vi "GeoData.vi"() -> ()   [LabVIEW 2017] (continued)
H1\n93203\t6029\tArvin\tCA\tKern County\tH1\n93250\t6029\tMc farland\tCA\tKern County\tH1\n93206\t6029\tButtonwillow\tCA\tKern County\tH1\n93384\t6029\tBakersfield\tCA\tKern County\tH1\n93502\t6029\tMojave\tCA\tKern County\tH1\n93255\t6029\tOnyx\tCA\tKern County\tH1\n93226\t6029\tGlennville\tCA\tKern County\tH1\n93528\t6029\tJohannesburg\tCA\tKern County\tH1\n93301\t6029\tBakersfield\tCA\tKern County\tH1\n93308\t6029\tBakersfield\tCA\tKern County\tH1\n93305\t6029\tBakersfield\tCA\tKern County\tH1\n93302\t6029\tBakersfield\tCA\tKern County\tH1\n93505\t6029\tCalifornia city\tCA\tKern County\tH1\n93561\t6029\tTehachapi\tCA\tKern County\tH1\n93461\t6029\tShandon\tCA\tKern County\tH1\n93268\t6029\tTaft\tCA\tKern County\tH1\n93241\t6029\tLamont\tCA\tKern County\tH1\n93263\t6029\tShafter\tCA\tKern County\tH1\n93518\t6029\tCaliente\tCA\tKern County\tH1\n93249\t6029\tLost hills\tCA\tKern County\tH1\n93303\t6029\tBakersfield\tCA\tKern County\tH1\n93222\t6029\tPine mountain club\tCA\tKern County\tH1\n93312\t6029\tBakersfield\tCA\tKern County\tH1\n93501\t6029\tMojave\tCA\tKern County\tH1\n93523\t6029\tEdwards\tCA\tKern County\tH1\n93240\t6029\tLake isabella\tCA\tKern County\tH1\n93238\t6029\tKernville\tCA\tKern County\tH1\n93251\t6029\tMc kittrick\tCA\tKern County\tH1\n93313\t6029\tBakersfield\tCA\tKern County\tH1\n93536\t6029\tLancaster\tCA\tKern County\tH1\n93516\t6029\tBoron\tCA\tKern County\tH1\n93219\t6029\tEarlimart\tCA\tKern County\tH1\n93224\t6029\tFellows\tCA\tKern County\tH1\n93252\t6029\tMaricopa\tCA\tKern County\tH1\n93554\t6029\tRandsburg\tCA\tKern County\tH1\n93309\t6029\tBakersfield\tCA\tKern County\tH1\n93387\t6029\tBakersfield\tCA\tKern County\tH1\n93524\t6029\tEdwards\tCA\tKern County\tH1\n93531\t6029\tKeene\tCA\tKern County\tH1\n93276\t6029\tTupman\tCA\tKern County\tH1\n93314\t6029\tBakersfield\tCA\tKern County\tH1\n93527\t6029\tInyokern\tCA\tKern County\tH1\n93225\t6029\tFrazier park\tCA\tKern County\tH1\n93280\t6029\tWasco\tCA\tKern County\tH1\n93389\t6029\tBakersfield\tCA\tKern County\tH1\n93239\t6031\tKettleman city\tCA\tKings County\tH1\n93266\t6031\tStratford\tCA\tKings County\tH1\n93656\t6031\tRiverdale\tCA\tKings County\tH1\n93274\t6031\tTulare\tCA\tKings County\tH1\n93246\t6031\tLemoore\tCA\tKings County\tH1\n93204\t6031\tAvenal\tCA\tKings County\tH1\n93230\t6031\tHanford\tCA\tKings County\tH1\n93631\t6031\tKingsburg\tCA\tKings County\tH1\n93212\t6031\tCorcoran\tCA\tKings County\tH1\n93202\t6031\tArmona\tCA\tKings County\tH1\n93232\t6031\tHanford\tCA\tKings County\tH1\n93245\t6031\tLemoore\tCA\tKings County\tH1\n93242\t6031\tLaton\tCA\tKings County\tH1\n95457\t6033\tLower lake\tCA\tLake County\tH1\n95423\t6033\tClearlake oaks\tCA\tLake County\tH1\n95424\t6033\tClearlake park\tCA\tLake County\tH1\n95451\t6033\tKelseyville\tCA\tLake County\tH1\n95467\t6033\tHidden valley lake\tCA\tLake County\tH1\n95485\t6033\tUpper lake\tCA\tLake County\tH1\n95422\t6033\tClearlake\tCA\tLake County\tH1\n95458\t6033\tLucerne\tCA\tLake County\tH1\n95453\t6033\tLakeport\tCA\tLake County\tH1\n95461\t6033\tMiddletown\tCA\tLake County\tH1\n95435\t6033\tFinley\tCA\tLake County\tH1\n95464\t6033\tNice\tCA\tLake County\tH1\n95443\t6033\tGlenhaven\tCA\tLake County\tH1\n95426\t6033\tCobb\tCA\tLake County\tH1\n95469\t6033\tPotter valley\tCA\tLake County\tH1\n95493\t6033\tWitter springs\tCA\tLake County\tH1\n96114\t6035\tJanesville\tCA\tLassen County\tH1\n96121\t6035\tMilford\tCA\tLassen County\tH1\n96128\t6035\tStandish\tCA\tLassen County\tH1\n96132\t6035\tTermo\tCA\tLassen County\tH1\n96136\t6035\tWendel\tCA\tLassen County\tH1\n96119\t6035\tMadeline\tCA\tLassen County\tH1\n96109\t6035\tDoyle\tCA\tLassen County\tH1\n96009\t6035\tBieber\tCA\tLassen County\tH1\n96127\t6035\tSusanville\tCA\tLassen County\tH1\n96117\t6035\tLitchfield\tCA\tLassen County\tH1\n96130\t6035\tSusanville\tCA\tLassen County\tH1\n96056\t6035\tMcarthur\tCA\tLassen County\tH1\n96068\t6035\tNubieber\tCA\tLassen County\tH1\n96137\t6035\tWestwood\tCA\tLassen County\tH1\n96113\t6035\tHerlong\tCA\tLassen County\tH1\n96123\t6035\tRavendale\tCA\tLassen County\tH1\n90013\t6037\tLos angeles\tCA\tLos Angeles County\tH1\n90232\t6037\tCulver city\tCA\tLos Angeles County\tH1\n90067\t6037\tLos angeles\tCA\tLos Angeles County\tH1\n90254\t6037\tHermosa beach\tCA\tLos Angeles County\tH1\n90305\t6037\tInglewood\tCA\tLos Angeles County\tH1\n90409\t6037\tSanta monica\tCA\tLos Angeles County\tH1\n90723\t6037\tParamount\tCA\tLos Angeles County\tH1\n90749\t6037\tCarson\tCA\tLos Angeles County\tH1\n90710\t6037\tHarbor city\tCA\tLos Angeles County\tH1\n90507\t6037\tTorrance\tCA\tLos Angeles County\tH1\n90043\t6037\tLos angeles\tCA\tLos Angeles County\tH1\n90059\t6037\tLos angeles\tCA\tLos Angeles County\tH1\n91101\t6037\tPasadena\tCA\tLos Angeles County\tH1\n91202\t6037\tGlendale\tCA\tLos Angeles County\tH1\n91008\t6037\tDuarte\tCA\tLos Angeles County\tH1\n91304\t6037\tCanoga park\tCA\tLos Angeles County\tH1\n91328\t6037\tNorthridge\tCA\tLos Angeles County\tH1\n91307\t6037\tWest hills\tCA\tLos Angeles County\tH1\n93560\t6037\tRosamond\tCA\tLos Angeles County\tH1\n91384\t6037\tCastaic\tCA\tLos Angeles County\tH1\n91405\t6037\tVan nuys\tCA\tLos Angeles County\tH1\n91345\t6037\tMission hills\tCA\tLos Angeles County\tH1\n91350\t6037\tSanta clarita\tCA\tLos Angeles County\tH1\n90670\t6037\tSanta fe springs\tCA\tLos Angeles County\tH1\n90660\t6037\tPico rivera\tCA\tLos Angeles County\tH1\n90638\t6037\tLa mirada\tCA\tLos Angeles County\tH1\n91711\t6037\tClaremont\tCA\tLos Angeles County\tH1\n91755\t6037\tMonterey park\tCA\tLos Angeles County\tH1\n91791\t6037\tWest covina\tCA\tLos Angeles County\tH1\n91770\t6037\tRosemead\tCA\tLos Angeles County\tH1\n91780\t6037\tTemple city\tCA\tLos Angeles County\tH1\n90051\t6037\tLos angeles\tCA\tLos Angeles County\tH1\n91025\t6037\tSierra madre\tCA\tLos Angeles County\tH1\n91778\t6037\tSan gabriel\tCA\tLos Angeles County\tH1\n91614\t6037\tStudio city\tCA\tLos Angeles County\tH1\n91066\t6037\tArcadia\tCA\tLos Angeles County\tH1\n91327\t6037\tNorthridge\tCA\tLos Angeles County\tH1\n93243\t6037\tLebec\tCA\tLos Angeles County\tH1\n91407\t6037\tVan nuys\tCA\tLos Angeles County\tH1\n90310\t6037\tInglewood\tCA\tLos Angeles County\tH1\n91603\t6037\tNorth hollywood\tCA\tLos Angeles County\tH1\n90306\t6037\tInglewood\tCA\tLos Angeles County\tH1\n91021\t6037\tMontrose\tCA\tLos Angeles County\tH1\n90822\t6037\tLong beach\tCA\tLos Angeles County\tH1\n91123\t6037\tPasadena\tCA\tLos Angeles County\tH1\n91129\t6037\tPasadena\tCA\tLos Angeles County\tH1\n91804\t6037\tAlhambra\tCA\tLos Angeles County\tH1\n90017\t6037\tLos angeles\tCA\tLos Angeles County\tH1\n90021\t6037\tLos angeles\tCA\tLos Angeles County\tH1\n90210\t6037\tBeverly hills\tCA\tLos Angeles County\tH1\n90071\t6037\tLos angeles\tCA\tLos Angeles County\tH1\n90266\t6037\tManhattan beach\tCA\tLos Angeles County\tH1\n90265\t6037\tMalibu\tCA\tLos Angeles County\tH1\n90401\t6037\tSanta monica\tCA\tLos Angeles County\tH1\n90503\t6037\tTorrance\tCA\tLos Angeles County\tH1\n90267\t6037\tManhattan beach\tCA\tLos Angeles County\tH1\n90505\t6037\tTorrance\tCA\tLos Angeles County\tH1\n90748\t6037\tWilmington\tCA\tLos Angeles County\tH1\n90039\t6037\tLos angeles\tCA\tLos Angeles County\tH1\n90033\t6037\tLos angeles\tCA\tLos Angeles County\tH1\n90065\t6037\tLos angeles\tCA\tLos Angeles County\tH1\n90058\t6037\tLos angeles\tCA\tLos Angeles County\tH1\n91016\t6037\tMonrovia\tCA\tLos Angeles County\tH1\n91030\t6037\tSouth pasadena\tCA\tLos Angeles County\tH1\n91105\t6037\tPasadena\tCA\tLos Angeles County\tH1\n91207\t6037\tGlendale\tCA\tLos Angeles County\tH1\n91343\t6037\tNorth hills\tCA\tLos Angeles County\tH1\n91605\t6037\tNorth hollywood\tCA\tLos Angeles County\tH1\n91601\t6037\tNorth hollywood\tCA\tLos Angeles County\tH1\n91504\t6037\tBurbank\tCA\tLos Angeles County\tH1\n93550\t6037\tPalmdale\tCA\tLos Angeles County\tH1\n93534\t6037\tLancaster\tCA\tLos Angeles County\tH1\n93552\t6037\tPalmdale\tCA\tLos Angeles County\tH1\n93553\t6037\tPearblossom\tCA\tLos Angeles County\tH1\n91387\t6037\tCanyon country\tCA\tLos Angeles County\tH1\n91386\t6037\tCanyon country\tCA\tLos Angeles County\tH1\n90604\t6037\tWhittier\tCA\tLos Angeles County\tH1\n90605\t6037\tWhittier\tCA\tLos Angeles County\tH1\n90606\t6037\tWhittier\tCA\tLos Angeles County\tH1\n91723\t6037\tCovina\tCA\tLos Angeles County\tH1\n91734\t6037\tEl monte\tCA\tLos Angeles County\tH1\n91750\t6037\tLa verne\tCA\tLos Angeles County\tH1\n91801\t6037\tAlhambra\tCA\tLos Angeles County\tH1\n91773\t6037\tSan dimas\tCA\tLos Angeles County\tH1\n91790\t6037\tWest covina\tCA\tLos Angeles County\tH1\n90052\t6037\tLos angeles\tCA\tLos Angeles County\tH1\n90840\t6037\tLong beach\tCA\tLos Angeles County\tH1\n91210\t6037\tGlendale\tCA\tLos Angeles County\tH1\n91322\t6037\tNewhall\tCA\tLos Angeles County\tH1\n91003\t6037\tAltadena\tCA\tLos Angeles County\tH1\n91310\t6037\tCastaic\tCA\tLos Angeles County\tH1\n93584\t6037\tLancaster\tCA\tLos Angeles County\tH1\n90408\t6037\tSanta monica\tCA\tLos Angeles County\tH1\n90734\t6037\tSan pedro\tCA\tLos Angeles County\tH1\n91226\t6037\tGlendale\tCA\tLos Angeles County\tH1\n91385\t6037\tValencia\tCA\tLos Angeles County\tH1\n91503\t6037\tBurbank\tCA\tLos Angeles County\tH1\n90506\t6037\tTorrance\tCA\tLos Angeles County\tH1\n90651\t6037\tNorwalk\tCA\tLos Angeles County\tH1\n90084\t6037\tLos angeles\tCA\tLos Angeles County\tH1\n91714\t6037\tCity of industry\tCA\tLos Angeles County\tH1\n91772\t6037\tRosemead\tCA\tLos Angeles County\tH1\n90662\t6037\tPico rivera\tCA\tLos Angeles County\tH1\n91899\t6037\tAlhambra\tCA\tLos Angeles County\tH1\n91329\t6037\tNorthridge\tCA\tLos Angeles County\tH1\n91522\t6037\tBurbank\tCA\tLos Angeles County\tH1\n91495\t6037\tSherman oaks\tCA\tLos Angeles County\tH1\n90012\t6037\tLos angeles\tCA\tLos Angeles County\tH1\n90019\t6037\tLos angeles\tCA\tLos Angeles County\tH1\n90024\t6037\tLos angeles\tCA\tLos Angeles County\tH1\n90005\t6037\tLos angeles\tCA\tLos Angeles County\tH1\n90010\t6037\tLos angeles\tCA\tLos Angeles County\tH1\n90023\t6037\tLos angeles\tCA\tLos Angeles County\tH1\n90231\t6037\tCulver city\tCA\tLos Angeles County\tH1\n90245\t6037\tEl segundo\tCA\tLos Angeles County\tH1\n90249\t6037\tGardena\tCA\tLos Angeles County\tH1\n90066\t6037\tLos angeles\tCA\tLos Angeles County\tH1\n90201\t6037\tBell gardens\tCA\tLos Angeles County\tH1\n90240\t6037\tDowney\tCA\tLos Angeles County\tH1\n90262\t6037\tLynwood\tCA\tLos Angeles County\tH1\n90091\t6037\tLos angeles\tCA\tLos Angeles County\tH1\n90275\t6037\tRancho palos verdes\tCA\tLos Angeles County\tH1\n90716\t6037\tHawaiian gardens\tCA\tLos Angeles County\tH1\n90745\t6037\tCarson\tCA\tLos Angeles County\tH1\n90701\t6037\tArtesia\tCA\tLos Angeles County\tH1\n90755\t6037\tSignal hill\tCA\tLos Angeles County\tH1\n90806\t6037\tLong beach\tCA\tLos Angeles County\tH1\n90036\t6037\tLos angeles\tCA\tLos Angeles County\tH1\n90038\t6037\tLos angeles\tCA\tLos Angeles County\tH1\n90040\t6037\tLos angeles\tCA\tLos Angeles County\tH1\n90032\t6037\tLos angeles\tCA\tLos Angeles County\tH1\n90049\t6037\tLos angeles\tCA\tLos Angeles County\tH1\n90061\t6037\tLos angeles\tCA\tLos Angeles County\tH1\n91020\t6037\tMontrose\tCA\tLos Angeles County\tH1\n91040\t6037\tSunland\tCA\tLos Angeles County\tH1\n91201\t6037\tGlendale\tCA\tLos Angeles County\tH1\n91301\t6037\tAgoura hills\tCA\tLos Angeles County\tH1\n91604\t6037\tStudio city\tCA\tLos Angeles County\tH1\n91606\t6037\tNorth hollywood\tCA\tLos Angeles County\tH1\n91609\t6037\tNorth hollywood\tCA\tLos Angeles County\tH1\n93543\t6037\tLittlerock\tCA\tLos Angeles County\tH1\n91361\t6037\tWestlake village\tCA\tLos Angeles County\tH1\n91381\t6037\tStevenson ranch\tCA\tLos Angeles County\tH1\n91390\t6037\tSanta clarita\tCA\tLos Angeles County\tH1\n91403\t6037\tSherman oaks\tCA\tLos Angeles County\tH1\n91352\t6037\tSun valley\tCA\tLos Angeles County\tH1\n91364\t6037\tWoodland hills\tCA\tLos Angeles County\tH1\n91423\t6037\tSherman oaks\tCA\tLos Angeles County\tH1\n91501\t6037\tBurbank\tCA\tLos Angeles County\tH1\n90650\t6037\tNorwalk\tCA\tLos Angeles County\tH1\n90609\t6037\tWhittier\tCA\tLos Angeles County\tH1\n91740\t6037\tGlendora\tCA\tLos Angeles County\tH1\n91745\t6037\tHacienda heights\tCA\tLos Angeles County\tH1\n91709\t6037\tChino hills\tCA\tLos Angeles County\tH1\n91731\t6037\tEl monte\tCA\tLos Angeles County\tH1\n91767\t6037\tPomona\tCA\tLos Angeles County\tH1\n91793\t6037\tWest covina\tCA\tLos Angeles County\tH1\n90714\t6037\tLakewood\tCA\tLos Angeles County\tH1\n91043\t6037\tTujunga\tCA\tLos Angeles County\tH1\n91117\t6037\tPasadena\tCA\tLos Angeles County\tH1\n93591\t6037\tPalmdale\tCA\tLos Angeles County\tH1\n90711\t6037\tLakewood\tCA\tLos Angeles County\tH1\n90060\t6037\tLos angeles\tCA\tLos Angeles County\tH1\n91341\t6037\tSan fernando\tCA\tLos Angeles County\tH1\n91346\t6037\tMission hills\tCA\tLos Angeles County\tH1\n91610\t6037\tToluca lake\tCA\tLos Angeles County\tH1\n93586\t6037\tLancaster\tCA\tLos Angeles County\tH1\n91305\t6037\tCanoga park\tCA\tLos Angeles County\tH1\n91222\t6037\tGlendale\tCA\tLos Angeles County\tH1\n91199\t6037\tPasadena\tCA\tLos Angeles County\tH1\n91496\t6037\tVan nuys\tCA\tLos Angeles County\tH1\n91612\t6037\tNorth hollywood\tCA\tLos Angeles County\tH1\n91523\t6037\tBurbank\tCA\tLos Angeles County\tH1\n91482\t6037\tVan nuys\tCA\tLos Angeles County\tH1\n90661\t6037\tPico rivera\tCA\tLos Angeles County\tH1\n91371\t6037\tWoodland hills\tCA\tLos Angeles County\tH1\n91185\t6037\tPasadena\tCA\tLos Angeles County\tH1\n90022\t6037\tLos angeles\tCA\tLos Angeles County\tH1\n90014\t6037\tLos angeles\tCA\tLos Angeles County\tH1\n90230\t6037\tCulver city\tCA\tLos Angeles County\tH1\n90239\t6037\tDowney\tCA\tLos Angeles County\tH1\n90247\t6037\tGardena\tCA\tLos Angeles County\tH1\n90241\t6037\tDowney\tCA\tLos Angeles County\tH1\n90248\t6037\tGardena\tCA\tLos Angeles County\tH1\n90213\t6037\tBeverly hills\tCA\tLos Angeles County\tH1\n90304\t6037\tInglewood\tCA\tLos Angeles County\tH1\n90274\t6037\tPalos verdes peninsula\tCA\tLos Angeles County\tH1\n90290\t6037\tTopanga\tCA\tLos Angeles County\tH1\n90405\t6037\tSanta monica\tCA\tLos Angeles County\tH1\n90732\t6037\tSan pedro\tCA\tLos Angeles County\tH1\n90713\t6037\tLakewood\tCA\tLos Angeles County\tH1\n90715\t6037\tLakewood\tCA\tLos Angeles County\tH1\n90804\t6037\tLong beach\tCA\tLos Angeles County\tH1\n90702\t6037\tArtesia\tCA\tLos Angeles County\tH1\n90047\t6037\tLos angeles\tCA\tLos Angeles County\tH1\n90064\t6037\tLos angeles\tCA\tLos Angeles County\tH1\n90063\t6037\tLos angeles\tCA\tLos Angeles County\tH1\n91006\t6037\tArcadia\tCA\tLos Angeles County\tH1\n90810\t6037\tLong beach\tCA\tLos Angeles County\tH1\n91001\t6037\tAltadena\tCA\tLos Angeles County\tH1\n91204\t6037\tGlendale\tCA\tLos Angeles County\tH1\n91115\t6037\tPasadena\tCA\tLos Angeles County\tH1\n91108\t6037\tSan marino\tCA\tLos Angeles County\tH1\n90002\t6037\tLos angeles\tCA\tLos Angeles County\tH1\n91206\t6037\tGlendale\tCA\tLos Angeles County\tH1\n91340\t6037\tSan fernando\tCA\tLos Angeles County\tH1\n91342\t6037\tSylmar\tCA\tLos Angeles County\tH1\n91208\t6037\tGlendale\tCA\tLos Angeles County\tH1\n91344\t6037\tGranada hills\tCA\tLos Angeles County\tH1\n91334\t6037\tPacoima\tCA\tLos Angeles County\tH1\n91617\t6037\tValley village\tCA\tLos Angeles County\tH1\n93532\t6037\tLake hughes\tCA\tLos Angeles County\tH1\n91351\t6037\tCanyon country\tCA\tLos Angeles County\tH1\n91436\t6037\tEncino\tCA\tLos Angeles County\tH1\n91502\t6037\tBurbank\tCA\tLos Angeles County\tH1\n90640\t6037\tMontebello\tCA\tLos Angeles County\tH1\n91733\t6037\tSouth el monte\tCA\tLos Angeles County\tH1\n91710\t6037\tChino\tCA\tLos Angeles County\tH1\n91748\t6037\tRowland heights\tCA\tLos Angeles County\tH1\n90009\t6037\tLos angeles\tCA\tLos Angeles County\tH1\n90202\t6037\tBell\tCA\tLos Angeles County\tH1\n91372\t6037\tCalabasas\tCA\tLos Angeles County\tH1\n91102\t6037\tPasadena\tCA\tLos Angeles County\tH1\n91118\t6037\tSan marino\tCA\tLos Angeles County\tH1\n91508\t6037\tBurbank\tCA\tLos Angeles County\tH1\n91769\t6037\tPomona\tCA\tLos Angeles County\tH1\n90095\t6037\tLos angeles\tCA\tLos Angeles County\tH1\n90607\t6037\tWhittier\tCA\tLos Angeles County\tH1\n90070\t6037\tLos angeles\tCA\tLos Angeles County\tH1\n90251\t6037\tHawthorne\tCA\tLos Angeles County\tH1\n93563\t6037\tValyermo\tCA\tLos Angeles County\tH1\n91046\t6037\tVerdugo city\tCA\tLos Angeles County\tH1\n90074\t6037\tLos angeles\tCA\tLos Angeles County\tH1\n90899\t6037\tLong beach\tCA\tLos Angeles County\tH1\n90639\t6037\tLa mirada\tCA\tLos Angeles County\tH1\n90833\t6037\tLong beach\tCA\tLos Angeles County\tH1\n90671\t6037\tSanta fe springs\tCA\tLos Angeles County\tH1\n90016\t6037\tLos angeles\tCA\tLos Angeles County\tH1\n90018\t6037\tLos angeles\tCA\tLos Angeles County\tH1\n90020\t6037\tLos angeles\tCA\tLos Angeles County\tH1\n90007\t6037\tLos angeles\tCA\tLos Angeles County\tH1\n90220\t6037\tCompton\tCA\tLos Angeles County\tH1\n90069\t6037\tWest hollywood\tCA\tLos Angeles County\tH1\n90303\t6037\tInglewood\tCA\tLos Angeles County\tH1\n90501\t6037\tTorrance\tCA\tLos Angeles County\tH1\n90295\t6037\tMarina del rey\tCA\tLos Angeles County\tH1\n90504\t6037\tTorrance\tCA\tLos Angeles County\tH1\n90042\t6037\tLos angeles\tCA\tLos Angeles County\tH1\n90034\t6037\tLos angeles\tCA\tLos Angeles County\tH1\n90815\t6037\tLong beach\tCA\tLos Angeles County\tH1\n90853\t6037\tLong beach\tCA\tLos Angeles County\tH1\n91024\t6037\tSierra madre\tCA\tLos Angeles County\tH1\n91042\t6037\tTujunga\tCA\tLos Angeles County\tH1\n91203\t6037\tGlendale\tCA\tLos Angeles County\tH1\n90003\t6037\tLos angeles\tCA\tLos Angeles County\tH1\n91306\t6037\tWinnetka\tCA\tLos Angeles County\tH1\n91302\t6037\tCalabasas\tCA\tLos Angeles County\tH1\n91330\t6037\tNorthridge\tCA\tLos Angeles County\tH1\n91506\t6037\tBurbank\tCA\tLos Angeles County\tH1\n91608\t6037\tUniversal city\tCA\tLos Angeles County\tH1\n93535\t6037\tLancaster\tCA\tLos Angeles County\tH1\n91367\t6037\tWoodland hills\tCA\tLos Angeles County\tH1\n91355\t6037\tValencia\tCA\tLos Angeles County\tH1\n90602\t6037\tWhittier\tCA\tLos Angeles County\tH1\n91722\t6037\tCovina\tCA\tLos Angeles County\tH1\n91744\t6037\tLa puente\tCA\tLos Angeles County\tH1\n91702\t6037\tAzusa\tCA\tLos Angeles County\tH1\n91747\t6037\tLa puente\tCA\tLos Angeles County\tH1\n91746\t6037\tLa puente\tCA\tLos Angeles County\tH1\n91754\t6037\tMonterey park\tCA\tLos Angeles County\tH1\n91768\t6037\tPomona\tCA\tLos Angeles County\tH1\n91765\t6037\tDiamond bar\tCA\tLos Angeles County\tH1\n90309\t6037\tInglewood\tCA\tLos Angeles County\tH1\n91209\t6037\tGlendale\tCA\tLos Angeles County\tH1\n91510\t6037\tBurbank\tCA\tLos Angeles County\tH1\n90637\t6037\tLa mirada\tCA\tLos Angeles County\tH1\n91802\t6037\tAlhambra\tCA\tLos Angeles County\tH1\n91416\t6037\tEncino\tCA\tLos Angeles County\tH1\n90086\t6037\tLos angeles\tCA\tLos Angeles County\tH1\n90093\t6037\tLos angeles\tCA\tLos Angeles County\tH1\n90308\t6037\tInglewood\tCA\tLos Angeles County\tH1\n91426\t6037\tEncino\tCA\tLos Angeles County\tH1\n91353\t6037\tSun valley\tCA\tLos Angeles County\tH1\n91771\t6037\tRosemead\tCA\tLos Angeles County\tH1\n90054\t6037\tLos angeles\tCA\tLos Angeles County\tH1\n91404\t6037\tVan nuys\tCA\tLos Angeles County\tH1\n91394\t6037\tGranada hills\tCA\tLos Angeles County\tH1\n91188\t6037\tPasadena\tCA\tLos Angeles County\tH1\n91716\t6037\tCity of industry\tCA\tLos Angeles County\tH1\n90846\t6037\tLong beach\tCA\tLos Angeles County\tH1\n91382\t6037\tSanta clarita\tCA\tLos Angeles County\tH1\n90011\t6037\tLos angeles\tCA\tLos Angeles County\tH1\n90004\t6037\tLos angeles\tCA\tLos Angeles County\tH1\n90008\t6037\tLos angeles\tCA\tLos Angeles County\tH1\n90026\t6037\tLos angeles\tCA\tLos Angeles County\tH1\n90028\t6037\tLos angeles\tCA\tLos Angeles County\tH1\n90068\t6037\tLos angeles\tCA\tLos Angeles County\tH1\n90260\t6037\tLawndale\tCA\tLos Angeles County\tH1\n90211\t6037\tBeverly hills\tCA\tLos Angeles County\tH1\n90075\t6037\tLos angeles\tCA\tLos Angeles County\tH1\n90278\t6037\tRedondo beach\tCA\tLos Angeles County\tH1\n90301\t6037\tInglewood\tCA\tLos Angeles County\tH1\n90302\t6037\tInglewood\tCA\tLos Angeles County\tH1\n90294\t6037\tVenice\tCA\tLos Angeles County\tH1\n90291\t6037\tVenice\tCA\tLos Angeles County\tH1\n90404\t6037\tSanta monica\tCA\tLos Angeles County\tH1\n90744\t6037\tWilmington\tCA\tLos Angeles County\tH1\n90746\t6037\tCarson\tCA\tLos Angeles County\tH1\n90510\t6037\tTorrance\tCA\tLos Angeles County\tH1\n90805\t6037\tLong beach\tCA\tLos Angeles County\tH1\n90703\t6037\tCerritos\tCA\tLos Angeles County\tH1\n90041\t6037\tLos angeles\tCA\tLos Angeles County\tH1\n90046\t6037\tLos angeles\tCA\tLos Angeles County\tH1\n90035\t6037\tLos angeles\tCA\tLos Angeles County\tH1\n91103\t6037\tPasadena\tCA\tLos Angeles County\tH1\n90813\t6037\tLong beach\tCA\tLos Angeles County\tH1\n90814\t6037\tLong beach\tCA\tLos Angeles County\tH1\n91107\t6037\tPasadena\tCA\tLos Angeles County\tH1\n91114\t6037\tPasadena\tCA\tLos Angeles County\tH1\n91106\t6037\tPasadena\tCA\tLos Angeles County\tH1\n90001\t6037\tLos angeles\tCA\tLos Angeles County\tH1\n91205\t6037\tGlendale\tCA\tLos Angeles County\tH1\n91335\t6037\tReseda\tCA\tLos Angeles County\tH1\n91602\t6037\tNorth hollywood\tCA\tLos Angeles County\tH1\n93063\t6037\tSimi valley\tCA\tLos Angeles County\tH1\n93536\t6037\tLancaster\tCA\tLos Angeles County\tH1\n93539\t6037\tLancaster\tCA\tLos Angeles County\tH1\n91362\t6037\tThousand oaks\tCA\tLos Angeles County\tH1\n91401\t6037\tVan nuys\tCA\tLos Angeles County\tH1\n91376\t6037\tAgoura hills\tCA\tLos Angeles County\tH1\n91392\t6037\tSylmar\tCA\tLos Angeles County\tH1\n92397\t6037\tWrightwood\tCA\tLos Angeles County\tH1\n90631\t6037\tLa habra\tCA\tLos Angeles County\tH1\n90601\t6037\tWhittier\tCA\tLos Angeles County\tH1\n91732\t6037\tEl monte\tCA\tLos Angeles County\tH1\n91786\t6037\tUpland\tCA\tLos Angeles County\tH1\n90083\t6037\tLos angeles\tCA\tLos Angeles County\tH1\n90508\t6037\tTorrance\tCA\tLos Angeles County\tH1\n90053\t6037\tLos angeles\tCA\tLos Angeles County\tH1\n91012\t6037\tLa canada flintridge\tCA\tLos Angeles County\tH1\n91396\t6037\tWinnetka\tCA\tLos Angeles County\tH1\n91031\t6037\tSouth pasadena\tCA\tLos Angeles County\tH1\n91109\t6037\tPasadena\tCA\tLos Angeles County\tH1\n93590\t6037\tPalmdale\tCA\tLos Angeles County\tH1\n90608\t6037\tWhittier\tCA\tLos Angeles County\tH1\n91788\t6037\tWalnut\tCA\tLos Angeles County\tH1\n90264\t6037\tMalibu\tCA\tLos Angeles County\tH1\n90261\t6037\tLawndale\tCA\tLos Angeles County\tH1\n90296\t6037\tPlaya del rey\tCA\tLos Angeles County\tH1\n91041\t6037\tSunland\tCA\tLos Angeles County\tH1\n91615\t6037\tNorth hollywood\tCA\tLos Angeles County\tH1\n91393\t6037\tNorth hills\tCA\tLos Angeles County\tH1\n90831\t6037\tLong beach\tCA\tLos Angeles County\tH1\n91023\t6037\tMount wilson\tCA\tLos Angeles County\tH1\n90076\t6037\tLos angeles\tCA\tLos Angeles County\tH1\n91224\t6037\tLa crescenta\tCA\tLos Angeles County\tH1\n91009\t6037\tDuarte\tCA\tLos Angeles County\tH1\n91507\t6037\tBurbank\tCA\tLos Angeles County\tH1\n91395\t6037\tMission hills\tCA\tLos Angeles County\tH1\n90223\t6037\tCompton\tCA\tLos Angeles County\tH1\n90307\t6037\tInglewood\tCA\tLos Angeles County\tH1\n93599\t6037\tPalmdale\tCA\tLos Angeles County\tH1\n90895\t6037\tCarson\tCA\tLos Angeles County\tH1\n90073\t6037\tLos angeles\tCA\tLos Angeles County\tH1\n91124\t6037\tPasadena\tCA\tLos Angeles County\tH1\n91125\t6037\tPasadena\tCA\tLos Angeles County\tH1\n91499\t6037\tVan nuys\tCA\tLos Angeles County\tH1\n90263\t6037\tMalibu\tCA\tLos Angeles County\tH1\n91470\t6037\tVan nuys\tCA\tLos Angeles County\tH1\n90610\t6037\tWhittier\tCA\tLos Angeles County\tH1\n90015\t6037\tLos angeles\tCA\tLos Angeles County\tH1\n90027\t6037\tLos angeles\tCA\tLos Angeles County\tH1\n90025\t6037\tLos angeles\tCA\tLos Angeles County\tH1\n90242\t6037\tDowney\tCA\tLos Angeles County\tH1\n90255\t6037\tHuntington park\tCA\tLos Angeles County\tH1\n90082\t6037\tLos angeles\tCA\tLos Angeles County\tH1\n90224\t6037\tCompton\tCA\tLos Angeles County\tH1\n90209\t6037\tBeverly hills\tCA\tLos Angeles County\tH1\n90072\t6037\tLos angeles\tCA\tLos Angeles County\tH1\n90293\t6037\tPlaya del rey\tCA\tLos Angeles County\tH1\n90402\t6037\tSanta monica\tCA\tLos Angeles County\tH1\n90280\t6037\tSouth gate\tCA\tLos Angeles County\tH1\n90502\t6037\tTorrance\tCA\tLos Angeles County\tH1\n90731\t6037\tSan pedro\tCA\tLos Angeles County\tH1\n90802\t6037\tLong beach\tCA\tLos Angeles County\tH1\n90706\t6037\tBellflower\tCA\tLos Angeles County\tH1\n90803\t6037\tLong beach\tCA\tLos Angeles County\tH1\n90707\t6037\tBellflower\tCA\tLos Angeles County\tH1\n90029\t6037\tLos angeles\tCA\tLos Angeles County\tH1\n90048\t6037\tLos angeles\tCA\tLos Angeles County\tH1\n90031\t6037\tLos angeles\tCA\tLos Angeles County\tH1\n90057\t6037\tLos angeles\tCA\tLos Angeles County\tH1\n90055\t6037\tLos angeles\tCA\tLos Angeles County\tH1\n91010\t6037\tDuarte\tCA\tLos Angeles County\tH1\n91017\t6037\tMonrovia\tCA\tLos Angeles County\tH1\n91104\t6037\tPasadena\tCA\tLos Angeles County\tH1\n91303\t6037\tCanoga park\tCA\tLos Angeles County\tH1\n91321\t6037\tNewhall\tCA\tLos Angeles County\tH1\n91325\t6037\tNorthridge\tCA\tLos Angeles County\tH1\n91214\t6037\tLa crescenta\tCA\tLos Angeles County\tH1\n91337\t6037\tReseda\tCA\tLos Angeles County\tH1\n91505\t6037\tBurbank\tCA\tLos Angeles County\tH1\n93544\t6037\tLlano\tCA\tLos Angeles County\tH1\n91380\t6037\tSanta clarita\tCA\tLos Angeles County\tH1\n91402\t6037\tPanorama city\tCA\tLos Angeles County\tH1\n91354\t6037\tValencia\tCA\tLos Angeles County\tH1\n91356\t6037\tTarzana\tCA\tLos Angeles County\tH1\n91411\t6037\tVan nuys\tCA\tLos Angeles County\tH1\n90623\t6037\tLa palma\tCA\tLos Angeles County\tH1\n91775\t6037\tSan gabriel\tCA\tLos Angeles County\tH1\n91789\t6037\tWalnut\tCA\tLos Angeles County\tH1\n91776\t6037\tSan gabriel\tCA\tLos Angeles County\tH1\n91766\t6037\tPomona\tCA\tLos Angeles County\tH1\n90087\t6037\tLos angeles\tCA\tLos Angeles County\tH1\n90078\t6037\tLos angeles\tCA\tLos Angeles County\tH1\n90050\t6037\tLos angeles\tCA\tLos Angeles County\tH1\n91309\t6037\tCanoga park\tCA\tLos Angeles County\tH1\n90801\t6037\tLong beach\tCA\tLos Angeles County\tH1\n91365\t6037\tWoodland hills\tCA\tLos Angeles County\tH1\n91357\t6037\tTarzana\tCA\tLos Angeles County\tH1\n91116\t6037\tPasadena\tCA\tLos Angeles County\tH1\n90099\t6037\tLos angeles\tCA\tLos Angeles County\tH1\n90081\t6037\tLos angeles\tCA\tLos Angeles County\tH1\n91611\t6037\tNorth hollywood\tCA\tLos Angeles County\tH1\n91184\t6037\tPasadena\tCA\tLos Angeles County\tH1\n91121\t6037\tPasadena\tCA\tLos Angeles County\tH1\n91521\t6037\tBurbank\tCA\tLos Angeles County\tH1\n91189\t6037\tPasadena\tCA\tLos Angeles County\tH1\n90509\t6037\tTorrance\tCA\tLos Angeles County\tH1\n91756\t6037\tMonterey park\tCA\tLos Angeles County\tH1\n91182\t6037\tPasadena\tCA\tLos Angeles County\tH1\n90844\t6037\tLong beach\tCA\tLos Angeles County\tH1\n90006\t6037\tLos angeles\tCA\tLos Angeles County\tH1\n90221\t6037\tCompton\tCA\tLos Angeles County\tH1\n90250\t6037\tHawthorne\tCA\tLos Angeles County\tH1\n90222\t6037\tCompton\tCA\tLos Angeles County\tH1\n90077\t6037\tLos angeles\tCA\tLos Angeles County\tH1\n90079\t6037\tLos angeles\tCA\tLos Angeles County\tH1\n90094\t6037\tPlaya vista\tCA\tLos Angeles County\tH1\n90212\t6037\tBeverly hills\tCA\tLos Angeles County\tH1\n90089\t6037\tLos angeles\tCA\tLos Angeles County\tH1\n90270\t6037\tMaywood\tCA\tLos Angeles County\tH1\n90272\t6037\tPacific palisades\tCA\tLos Angeles County\tH1\n90277\t6037\tRedondo beach\tCA\tLos Angeles County\tH1\n90292\t6037\tMarina del rey\tCA\tLos Angeles County\tH1\n90403\t6037\tSanta monica\tCA\tLos Angeles County\tH1\n90712\t6037\tLakewood\tCA\tLos Angeles County\tH1\n90717\t6037\tLomita\tCA\tLos Angeles County\tH1\n90037\t6037\tLos angeles\tCA\tLos Angeles County\tH1\n90044\t6037\tLos angeles\tCA\tLos Angeles County\tH1\n90045\t6037\tLos angeles\tCA\tLos Angeles County\tH1\n90062\t6037\tLos angeles\tCA\tLos Angeles County\tH1\n90056\t6037\tLos angeles\tCA\tLos Angeles County\tH1\n91007\t6037\tArcadia\tCA\tLos Angeles County\tH1\n90807\t6037\tLong beach\tCA\tLos Angeles County\tH1\n90808\t6037\tLong beach\tCA\tLos Angeles County\tH1\n91011\t6037\tLa canada flintridge\tCA\tLos Angeles County\tH1\n91311\t6037\tChatsworth\tCA\tLos Angeles County\tH1\n91324\t6037\tNorthridge\tCA\tLos Angeles County\tH1\n91326\t6037\tPorter ranch\tCA\tLos Angeles County\tH1\n91316\t6037\tEncino\tCA\tLos Angeles County\tH1\n91331\t6037\tPacoima\tCA\tLos Angeles County\tH1\n91607\t6037\tValley village\tCA\tLos Angeles County\tH1\n93510\t6037\tActon\tCA\tLos Angeles County\tH1\n93551\t6037\tPalmdale\tCA\tLos Angeles County\tH1\n91413\t6037\tSherman oaks\tCA\tLos Angeles County\tH1\n91406\t6037\tVan nuys\tCA\tLos Angeles County\tH1\n91409\t6037\tVan nuys\tCA\tLos Angeles County\tH1\n90603\t6037\tWhittier\tCA\tLos Angeles County\tH1\n90630\t6037\tCypress\tCA\tLos Angeles County\tH1\n90652\t6037\tNorwalk\tCA\tLos Angeles County\tH1\n91741\t6037\tGlendora\tCA\tLos Angeles County\tH1\n91706\t6037\tBaldwin park\tCA\tLos Angeles County\tH1\n91724\t6037\tCovina\tCA\tLos Angeles County\tH1\n91715\t6037\tCity of industry\tCA\tLos Angeles County\tH1\n91792\t6037\tWest covina\tCA\tLos Angeles County\tH1\n91803\t6037\tAlhambra\tCA\tLos Angeles County\tH1\n90733\t6037\tSan pedro\tCA\tLos Angeles County\tH1\n91333\t6037\tPacoima\tCA\tLos Angeles County\tH1\n91313\t6037\tChatsworth\tCA\tLos Angeles County\tH1\n91221\t6037\tGlendale\tCA\tLos Angeles County\tH1\n91408\t6037\tVan nuys\tCA\tLos Angeles County\tH1\n91308\t6037\tWest hills\tCA\tLos Angeles County\tH1\n90406\t6037\tSanta monica\tCA\tLos Angeles County\tH1\n90809\t6037\tLong beach\tCA\tLos Angeles County\tH1\n91412\t6037\tPanorama city\tCA\tLos Angeles County\tH1\n90832\t6037\tLong beach\tCA\tLos Angeles County\tH1\n91225\t6037\tGlendale\tCA\tLos Angeles County\tH1\n91077\t6037\tArcadia\tCA\tLos Angeles County\tH1\n91126\t6037\tPasadena\tCA\tLos Angeles County\tH1\n90030\t6037\tLos angeles\tCA\tLos Angeles County\tH1\n91383\t6037\tSanta clarita\tCA\tLos Angeles County\tH1\n90747\t6037\tCarson\tCA\tLos Angeles County\tH1\n90704\t6037\tAvalon\tCA\tLos Angeles County\tH1\n91896\t6037\tAlhambra\tCA\tLos Angeles County\tH1\n90090\t6037\tDodgertown\tCA\tLos Angeles County\tH1\n93639\t6039\tMadera\tCA\tMadera County\tH1\n93720\t6039\tFresno\tCA\tMadera County\tH1\n93669\t6039\tWishon\tCA\tMadera County\tH1\n93626\t6039\tFriant\tCA\tMadera County\tH1\n93620\t6039\tDos palos\tCA\tMadera County\tH1\n93645\t6039\tO neals\tCA\tMadera County\tH1\n93630\t6039\tKerman\tCA\tMadera County\tH1\n93637\t6039\tMadera\tCA\tMadera County\tH1\n93644\t6039\tOakhurst\tCA\tMadera County\tH1\n93614\t6039\tCoarsegold\tCA\tMadera County\tH1\n93602\t6039\tAuberry\tCA\tMadera County\tH1\n93622\t6039\tFirebaugh\tCA\tMadera County\tH1\n93636\t6039\tMadera\tCA\tMadera County\tH1\n93643\t6039\tNorth fork\tCA\tMadera County\tH1\n93604\t6039\tBass lake\tCA\tMadera County\tH1\n93601\t6039\tAhwahnee\tCA\tMadera County\tH1\n93610\t6039\tChowchilla\tCA\tMadera County\tH1\n93638\t6039\tMadera\tCA\tMadera County\tH1\n93653\t6039\tRaymond\tCA\tMadera County\tH1\n94979\t6041\tSan anselmo\tCA\tMarin County\tH1\n94924\t6041\tBolinas\tCA\tMarin County\tH1\n94963\t6041\tSan geronimo\tCA\tMarin County\tH1\n94929\t6041\tDillon beach\tCA\tMarin County\tH1\n94964\t6041\tSan quentin\tCA\tMarin County\tH1\n94950\t6041\tOlema\tCA\tMarin County\tH1\n94912\t6041\tSan rafael\tCA\tMarin County\tH1\n94938\t6041\tLagunitas\tCA\tMarin County\tH1\n94978\t6041\tFairfax\tCA\tMarin County\tH1\n94913\t6041\tSan rafael\tCA\tMarin County\tH1\n94901\t6041\tSan rafael\tCA\tMarin County\tH1\n94925\t6041\tCorte madera\tCA\tMarin County\tH1\n94930\t6041\tFairfax\tCA\tMarin County\tH1\n94947\t6041\tNovato\tCA\tMarin County\tH1\n94965\t6041\tSausalito\tCA\tMarin County\tH1\n94973\t6041\tWoodacre\tCA\tMarin County\tH1\n94948\t6041\tNovato\tCA\tMarin County\tH1\n94970\t6041\tStinson beach\tCA\tMarin County\tH1\n94949\t6041\tNovato\tCA\tMarin County\tH1\n94966\t6041\tSausalito\tCA\tMarin County\tH1\n94933\t6041\tForest knolls\tCA\tMarin County\tH1\n94940\t6041\tMarshall\tCA\tMarin County\tH1\n94952\t6041\tPetaluma\tCA\tMarin County\tH1\n94915\t6041\tSan rafael\tCA\tMarin County\tH1\n94942\t6041\tMill valley\tCA\tMarin County\tH1\n94976\t6041\tCorte madera\tCA\tMarin County\tH1\n94974\t6041\tSan quentin\tCA\tMarin County\tH1\n94904\t6041\tGreenbrae\tCA\tMarin County\tH1\n94939\t6041\tLarkspur\tCA\tMarin County\tH1\n94945\t6041\tNovato\tCA\tMarin County\tH1\n94960\t6041\tSan anselmo\tCA\tMarin County\tH1\n94957\t6041\tRoss\tCA\tMarin County\tH1\n94977\t6041\tLarkspur\tCA\tMarin County\tH1\n94903\t6041\tSan rafael\tCA\tMarin County\tH1\n94920\t6041\tBelvedere tiburon\tCA\tMarin County\tH1\n94941\t6041\tMill valley\tCA\tMarin County\tH1\n94956\t6041\tPoint reyes station\tCA\tMarin County\tH1\n94937\t6041\tInverness\tCA\tMarin County\tH1\n94971\t6041\tTomales\tCA\tMarin County\tH1\n94946\t6041\tNicasio\tCA\tMarin County\tH1\n94914\t6041\tKentfield\tCA\tMarin County\tH1\n95369\t6043\tSnelling\tCA\tMariposa County\tH1\n95311\t6043\tCoulterville\tCA\tMariposa County\tH1\n95345\t6043\tMidpines\tCA\tMariposa County\tH1\n95306\t6043\tCatheys valley\tCA\tMariposa County\tH1\n95338\t6043\tMariposa\tCA\tMariposa County\tH1\n93623\t6043\tFish camp\tCA\tMariposa County\tH1\n95321\t6043\tGroveland\tCA\tMariposa County\tH1\n95389\t6043\tYosemite national park\tCA\tMariposa County\tH1\n95325\t6043\tHornitos\tCA\tMariposa County\tH1\n95329\t6043\tLa grange\tCA\tMariposa County\tH1\n95318\t6043\tEl portal\tCA\tMariposa County\tH1\n93601\t6043\tAhwahnee\tCA\tMariposa County\tH1\n93653\t6043\tRaymond\tCA\tMariposa County\tH1\n95490\t6045\tWillits\tCA\tMendocino County\tH1\n95410\t6045\tAlbion\tCA\tMendocino County\tH1\n95460\t6045\tMendocino\tCA\tMendocino County\tH1\n95429\t6045\tDos rios\tCA\tMendocino County\tH1\n95418\t6045\tCalpella\tCA\tMendocino County\tH1\n95449\t6045\tHopland\tCA\tMendocino County\tH1\n95459\t6045\tManchester\tCA\tMendocino County\tH1\n95494\t6045\tYorkville\tCA\tMendocino County\tH1\n95428\t6045\tCovelo\tCA\tMendocino County\tH1\n95420\t6045\tCaspar\tCA\tMendocino County\tH1\n95432\t6045\tElk\tCA\tMendocino County\tH1\n95589\t6045\tWhitethorn\tCA\tMendocino County\tH1\n95468\t6045\tPoint arena\tCA\tMendocino County\tH1\n95542\t6045\tGarberville\tCA\tMendocino County\tH1\n95437\t6045\tFort bragg\tCA\tMendocino County\tH1\n95481\t6045\tTalmage\tCA\tMendocino County\tH1\n95463\t6045\tNavarro\tCA\tMendocino County\tH1\n95482\t6045\tUkiah\tCA\tMendocino County\tH1\n95454\t6045\tLaytonville\tCA\tMendocino County\tH1\n95427\t6045\tComptche\tCA\tMendocino County\tH1\n95470\t6045\tRedwood valley\tCA\tMendocino County\tH1\n95456\t6045\tLittle river\tCA\tMendocino County\tH1\n95585\t6045\tLeggett\tCA\tMendocino County\tH1\n95445\t6045\tGualala\tCA\tMendocino County\tH1\n95417\t6045\tBranscomb\tCA\tMendocino County\tH1\n95587\t6045\tPiercy\tCA\tMendocino County\tH1\n95488\t6045\tWestport\tCA\tMendocino County\tH1\n95466\t6045\tPhilo\tCA\tMendocino County\tH1\n95415\t6045\tBoonville\tCA\tMendocino County\tH1\n95469\t6045\tPotter valley\tCA\tMendocino County\tH1\n95340\t6047\tMerced\tCA\tMerced County\tH1\n95348\t6047\tMerced\tCA\tMerced County\tH1\n95369\t6047\tSnelling\tCA\tMerced County\tH1\n95374\t6047\tStevinson\tCA\tMerced County\tH1\n95333\t6047\tLe grand\tCA\tMerced County\tH1\n95360\t6047\tNewman\tCA\tMerced County\tH1\n95312\t6047\tCressey\tCA\tMerced County\tH1\n93620\t6047\tDos palos\tCA\tMerced County\tH1\n95388\t6047\tWinton\tCA\tMerced County\tH1\n95315\t6047\tDelhi\tCA\tMerced County\tH1\n95341\t6047\tMerced\tCA\tMerced County\tH1\n95316\t6047\tDenair\tCA\tMerced County\tH1\n95344\t6047\tMerced\tCA\tMerced County\tH1\n95343\t6047\tMerced\tCA\tMerced County\tH1\n93635\t6047\tLos banos\tCA\tMerced County\tH1\n95322\t6047\tGustine\tCA\tMerced County\tH1\n95324\t6047\tHilmar\tCA\tMerced County\tH1\n95334\t6047\tLivingston\tCA\tMerced County\tH1\n95303\t6047\tBallico\tCA\tMerced County\tH1\n95380\t6047\tTurlock\tCA\tMerced County\tH1\n95301\t6047\tAtwater\tCA\tMerced County\tH1\n95317\t6047\tEl nido\tCA\tMerced County\tH1\n93661\t6047\tSanta rita park\tCA\tMerced County\tH1\n93622\t6047\tFirebaugh\tCA\tMerced County\tH1\n93610\t6047\tChowchilla\tCA\tMerced County\tH1\n95365\t6047\tPlanada\tCA\tMerced County\tH1\n93665\t6047\tSouth dos palos\tCA\tMerced County\tH1\n96134\t6049\tTulelake\tCA\tModoc County\tH1\n96104\t6049\tCedarville\tCA\tModoc County\tH1\n96112\t6049\tFort bidwell\tCA\tModoc County\tH1\n96006\t6049\tAdin\tCA\tModoc County\tH1\n96115\t6049\tLake city\tCA\tModoc County\tH1\n96101\t6049\tAlturas\tCA\tModoc County\tH1\n96015\t6049\tCanby\tCA\tModoc County\tH1\n96054\t6049\tLookout\tCA\tModoc County\tH1\n96116\t6049\tLikely\tCA\tModoc County\tH1\n96056\t6049\tMcarthur\tCA\tModoc County\tH1\n96108\t6049\tDavis creek\tCA\tModoc County\tH1\n96110\t6049\tEagleville\tCA\tModoc County\tH1\n93546\t6051\tMammoth lakes\tCA\tMono County\tH1\n93529\t6051\tJune lake\tCA\tMono County\tH1\n93512\t6051\tBenton\tCA\tMono County\tH1\n93517\t6051\tBridgeport\tCA\tMono County\tH1\n96107\t6051\tColeville\tCA\tMono County\tH1\n93541\t6051\tLee vining\tCA\tMono County\tH1\n93514\t6051\tBishop\tCA\tMono County\tH1\n96133\t6051\tTopaz\tCA\tMono County\tH1\n93426\t6053\tBradley\tCA\tMonterey County\tH1\n93923\t6053\tCarmel\tCA\tMonterey County\tH1\n93960\t6053\tSoledad\tCA\tMonterey County\tH1\n95004\t6053\tAromas\tCA\tMonterey County\tH1\n93922\t6053\tCarmel\tCA\tMonterey County\tH1\n93921\t6053\tCarmel by the sea\tCA\tMonterey County\tH1\n93450\t6053\tSan ardo\tCA\tMonterey County\tH1\n93933\t6053\tMarina\tCA\tMonterey County\tH1\n93924\t6053\tCarmel valley\tCA\tMonterey County\tH1\n93902\t6053\tSalinas\tCA\tMonterey County\tH1\n93942\t6053\tMonterey\tCA\tMonterey County\tH1\n93943\t6053\tMonterey\tCA\tMonterey County\tH1\n93925\t6053\tChualar\tCA\tMonterey County\tH1\n93915\t6053\tSalinas\tCA\tMonterey County\tH1\n93940\t6053\tMonterey\tCA\tMonterey County\tH1\n93927\t6053\tGreenfield\tCA\tMonterey County\tH1\n93955\t6053\tSeaside\tCA\tMonterey County\tH1\n95076\t6053\tWatsonville\tCA\tMonterey County\tH1\n93944\t6053\tMonterey\tCA\tMonterey County\tH1\n93930\t6053\tKing city\tCA\tMonterey County\tH1\n93950\t6053\tPacific grove\tCA\tMonterey County\tH1\n93451\t6053\tSan miguel\tCA\tMonterey County\tH1\n93908\t6053\tSalinas\tCA\tMonterey County\tH1\n93906\t6053\tSalinas\tCA\tMonterey County\tH1\n93928\t6053\tJolon\tCA\tMonterey County\tH1\n93901\t6053\tSalinas\tCA\tMonterey County\tH1\n93905\t6053\tSalinas\tCA\tMonterey County\tH1\n93926\t6053\tGonzales\tCA\tMonterey County\tH1\n93954\t6053\tSan lucas\tCA\tMonterey County\tH1\n93210\t6053\tCoalinga\tCA\tMonterey County\tH1\n93907\t6053\tSalinas\tCA\tMonterey County\tH1\n93912\t6053\tSalinas\tCA\tMonterey County\tH1\n93953\t6053\tPebble beach\tCA\tMonterey County\tH1\n95012\t6053\tCastroville\tCA\tMonterey County\tH1\n93920\t6053\tBig sur\tCA\tMonterey County\tH1\n95039\t6053\tMoss landing\tCA\tMonterey County\tH1\n93962\t6053\tSpreckels\tCA\tMonterey County\tH1\n93932\t6053\tLockwood\tCA\tMonterey County\tH1\n94574\t6055\tSaint helena\tCA\tNapa County\tH1\n94515\t6055\tCalistoga\tCA\tNapa County\tH1\n94581\t6055\tNapa\tCA\tNapa County\tH1\n94599\t6055\tYountville\tCA\tNapa County\tH1\n94508\t6055\tAngwin\tCA\tNapa County\tH1\n94558\t6055\tNapa\tCA\tNapa County\tH1\n94503\t6055\tAmerican canyon\tCA\tNapa County\tH1\n94576\t6055\tDeer park\tCA\tNapa County\tH1\n94567\t6055\tPope valley\tCA\tNapa County\tH1\n94573\t6055\tRutherford\tCA\tNapa County\tH1\n95476\t6055\tSonoma\tCA\tNapa County\tH1\n95461\t6055\tMiddletown\tCA\tNapa County\tH1\n94559\t6055\tNapa\tCA\tNapa County\tH1\n94591\t6055\tVallejo\tCA\tNapa County\tH1\n94534\t6055\tFairfield\tCA\tNapa County\tH1\n94562\t6055\tOakville\tCA\tNapa County\tH1\n96162\t6057\tTruckee\tCA\tNevada County\tH1\n95946\t6057\tPenn valley\tCA\tNevada County\tH1\n95977\t6057\tSmartsville\tCA\tNevada County\t
